vi "ZeroMQ_Create.vi"(0 "reference in":refnum<class "ZeroMQ.lvclass">, 1 "Serializer":refnum<class "Serializer.lvclass">, 2 "IP address":string, 3 "Port":string, 4 "Executor":refnum<class "Executer.lvclass">, 5 "error in (no error)":errorcluster) -> (14 "reference out":refnum<class "ZeroMQ.lvclass">, 19 "error out":errorcluster)   [LabVIEW 2018, in "ZeroMQ.lvclass"]
doc: "This VI will create a communication class, for recieving messages from the other end, calling the executor to execute the methodand reutn the ouput back onto a message.\nIn this case ZeroMQ is the communication used."
uses:
  ZeroMQ.lvclass
  C:/VIT/VIT-Reuse/Examples/RemoteLabviewInterface/Communication/Communication_class/Communication.lvclass
  Executer_class/Executer.lvclass
  Serializers/Serializer_class/Serializer.lvclass
  Communication_class/Communication.lvclass
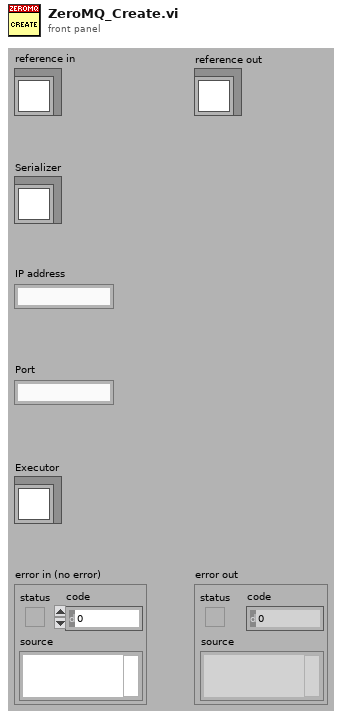
[diagram p1: front panel]
types:
  T1 = typedef "ZeroMQ.lvclass/ObjectAttributes.ctl" = cluster{"IP":string, "Port":string}
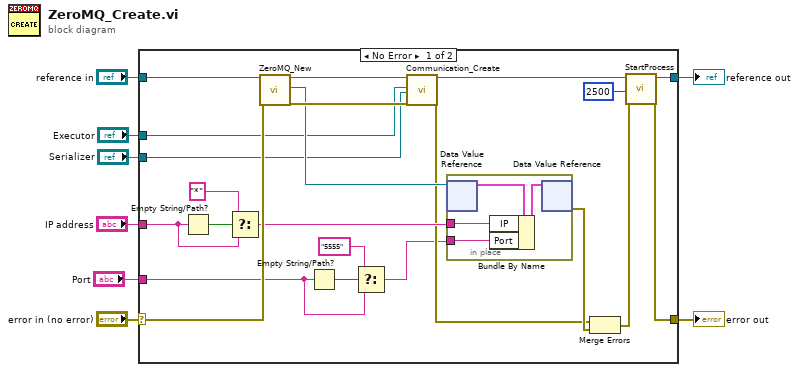
[diagram p0: block diagram]
diagram:
  n1 = case shown="No Error" "error in (no error)" {
    selector: "error in (no error)" -> [w29 w36]
    tunnel: [w21 w36] -> w7
    tunnel: "reference in" -> [w30 w35]
    tunnel: [w23 w35] -> w5
    tunnel: "IP address" -> [w18 _]
    tunnel: "Executor" -> [w15 _]
    tunnel: "Port" -> [w11 _]
    tunnel: "Serializer" -> [w9 _]
    frame No Error {
      n2 = Empty String/Path?(string/path=w18) -> (empty?=w19:bool)
      n3 = Select(t="*", s=w19, f=w18) -> (s? t:f=w17:string)
      n4 = call "ZeroMQ_New.vi"("reference in"=w30, "error in (no error)"=w29) -> ("reference out"=w27:refnum<class "ZeroMQ.lvclass">, "DVRRefOut"=w25:refnum<data-value>, "error out"=w26:errorcluster)  [unwired: 14 in, 1 out]
      n5 = Empty String/Path?(string/path=w11) -> (empty?=w13:bool)
      n6 = Select(t="5555", s=w13, f=w11) -> (s? t:f=w10:string)
      n7 = call "Communication_Create.vi"("reference in"=w27, "Executer"=w15, "Serializer"=w9, "error in (no error)"=w26) -> ("reference out"=w24:refnum<class "ZeroMQ.lvclass">, "error out"=w16:errorcluster)  [unwired: 14 in]
      n8 = in-place {
        in-place-border: w17 -> [w32]
        in-place-border: w10 -> [w31]
        n9 = in-place-dvr #1(w25) -> (w33:T1)  [unwired: 1 out]
        n10 = Bundle By Name(cluster=w33, "IP"=w32, "Port"=w31) -> (w34:T1)
        n11 = in-place-dvr #1(w34) -> (w28:errorcluster)  [unwired: 1 out]
      }
      n12 = Merge Errors(w16, w28) -> (w22:errorcluster)
      n13 = call "StartProcess.vi"("reference in"=w24, "ms timeout (-1)"=2500, "error in (no error)"=w22) -> ("reference out"=w23:refnum<class "ZeroMQ.lvclass">, "error out"=w21:errorcluster)  [unwired: 13 in, 2 out]
    }
    frame Error {
    }
  }
  "error out" <- w7
  "reference out" <- w5
